vi "Exponential Prediction.vi"() -> ()   [LabVIEW 2023]
doc: "This example shows how to forecast the future values of a univariate time series based on exponential smoothing with the TSA Exponential Prediction VI.\n\n<b>Instructions:</b>\n1) Run this VI.\n2) Compare the predicted sales record and real sales record."
uses:
  <vilib>/addons/Time Series Analysis/Utilities.llb/TSA Data.ctl
  <vilib>/addons/Time Series Analysis/Modeling and Prediction.llb/TSA Exponential Prediction (Array).vi
  <vilib>/addons/_Advanced Signal Processing/NI_AdvSigProcTSA.lvlib
panel:
  in  "stop":bool
  in  "Season Type":u16(ring) items=["Multiplicative", "Additive"]
  in  "Season period":i32=4
  in  "Exponential factors":cluster{"Level":dbl, "Trend":dbl, "Season":dbl}={"Level"=0.01, "Trend"=0.6, "Season"=0.9} {"Season" min=0.0 max=1.0 step=0.1; "Trend" min=0.0 max=1.0 step=0.1; "Level" min=0.0 max=1.0 step=0.1}
  in  "Exponential Type":u16(ring)=2 items=["Single", "Double", "Triple"]
  out "Sales Record":dbl[][](graph)
  in  "Number of predictions":i32=8
  # "Overview: Shows how to forecast the future values of a univariate time series based on exponential smoothing with the TSA Exponential Prediction VI.\nRequirements: LabVIEW Full Development System, Advanced Signal Processing Toolkit\nInstructions: \n1. Run this VI.\n2. Compare the predicted sales record and real sales record.\n3. Click Stop to stop the VI."
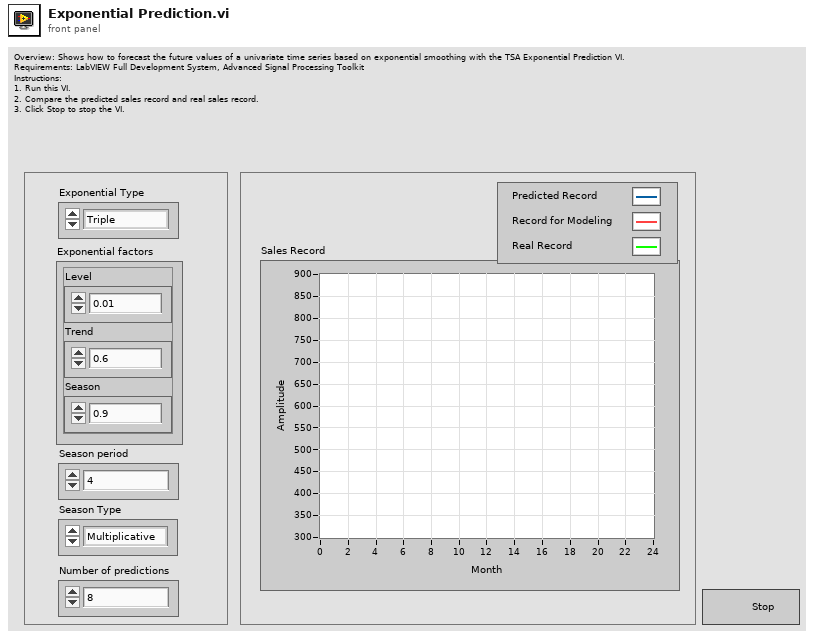
[diagram p1: front panel]
types:
  T1 = typedef "NI_AdvSigProcTSA.lvlib/TSA Data.ctl" = u16
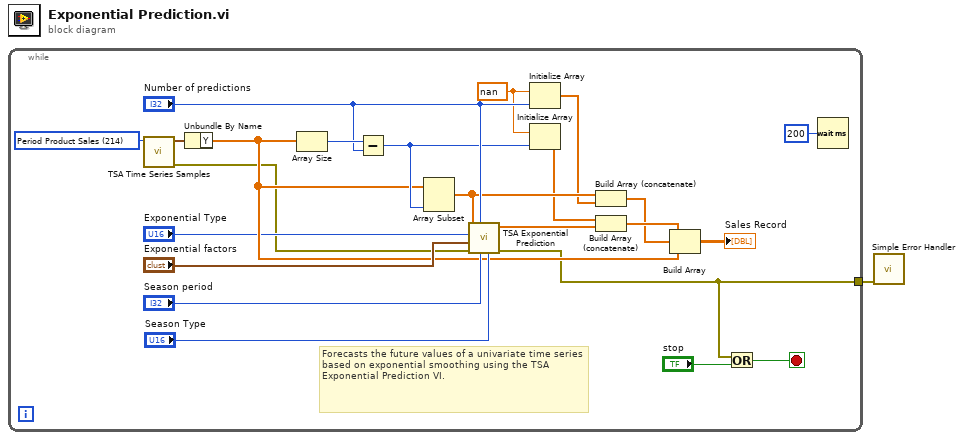
[diagram p0: block diagram]
diagram:
  n1 = while {
    tunnel: [w3] -> w1
    stop <- w9 stop-if-true
    w4 = T1 214 items=["Kobe Earthquake"=201, "EEG"=210, "Bearing Vibration (simulated)"=211, "Period Product Sales"=214, "Beam Vibration (nonlinear)"=217, "Beam Vibration (linear)"=218, "Signal With Echo"=219, "Engine Knocking"=220, "Power Line"=221, "-"=200, "Beam Deflections (multivariate)"=207, "Structure Vibration (multivariate)"=208, "Human MEG (multivariate)"=222] ("data")
    w20 = nan ("element")
    # "Forecasts the future values of a univariate time series based on exponential smoothing using the TSA Exponential Prediction VI."
    n2 = call <vilib>:"TSA Time Series Samples.vi"("data"=w4) -> ("error out"=w2:errorcluster, "univariate time series"=w16:waveform(dbl))  [unwired: 1 in, 8 out]
    n3 = Unbundle By Name(w16) -> ("Y"=w6:dbl[])
    n4 = Array Size(array=w6) -> (size(s)=w23:i32)
    n5 = Subtract(x=w23, y="Number of predictions") -> (x-y=w19:i32)
    n6 = Array Subset(array=w6, length=w19) -> (w14:dbl[])  [unwired: 1 in]
    n7 = call-poly <vilib>:"TSA Exponential Prediction.vi"("season type"="Season Type", "season period"="Season period", "number of points"="Number of predictions", "error in (no error)"=w2, "exponential factors"="Exponential factors", "exponential type"="Exponential Type", "Xt"=w14) -> ("error out"=w3:errorcluster, "predicted series"=w22:dbl[])  [unwired: 3 out]
    n8 = Initialize Array(w20, "Number of predictions") -> (w7:dbl[])
    n9 = Initialize Array(w20, w19) -> (w12:dbl[])
    n10 = Build Array (concatenate)(w14, w7) -> (w17:dbl[])
    n11 = Build Array (concatenate)(w12, w22) -> (w18:dbl[])
    n12 = Build Array(w18, w17, w6) -> (→"Sales Record":dbl[][])
    n13 = Or(x=w3, y="stop") -> (x .or. y?=w9:bool)
    n14 = Wait (ms)(milliseconds to wait=u32 200 ("millisecond multiple")) -> ()  [unwired: 1 out]
  }
  n15 = call <vilib>:"Simple Error Handler.vi"("error in (no error)"=w1) -> ()  [unwired: 1 in, 8 out]
